vi "add set current(SubVI).vi"() -> (1 "ok or cancel":bool=TRUE, 2 "连接的字符串":string)   [LabVIEW 2019, in "Add Seq.lvlib"]
uses:
  Add Seq.lvlib
panel:
  in  "Frequency(Hz)\n(-1表示不更改频率）":dbl=-1.0 format="%#_13g"
  in  "Current Amplitude(mA)":dbl
  in  "cancel":bool
  in  "ok":bool
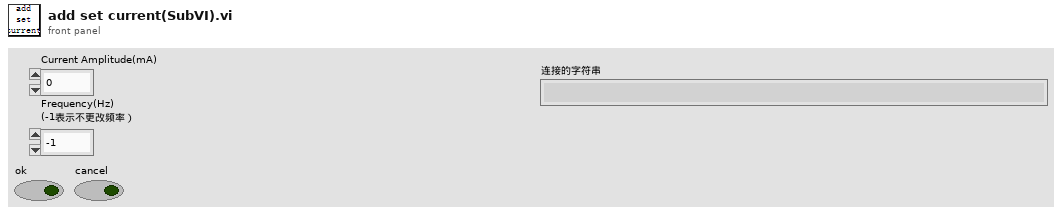
[diagram p1: front panel]
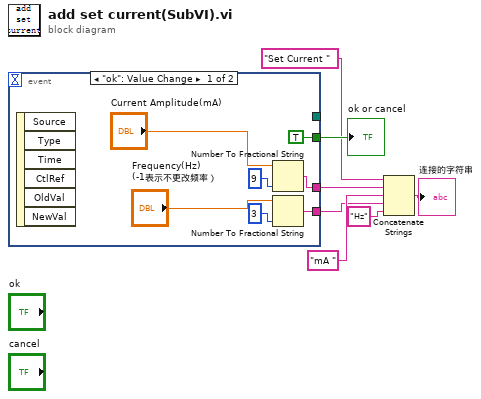
[diagram p0: block diagram]
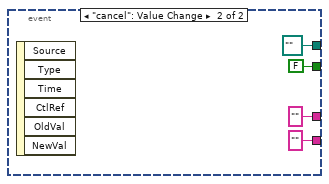
[diagram p2: hidden frame]
diagram:
  n1 = event shown="[0] \"ok\": Value Change" {
    selector: _ -> [_ _]
    dyn-events: _ -> [_ _]
    timeout: _ -> [_ _]
    tunnel: [_ path "" ("path")] -> _
    tunnel: [TRUE FALSE] -> w5
    tunnel: [w11 ""] -> w3
    tunnel: [w8 ""] -> w1
    event "ok": Value Change {
      n2 = event-data() -> ()  [unwired: 1 in, 6 out]
      n3 = Number To Fractional String(number="Current Amplitude(mA)", precision (6)=i16 9 ("精度(6)")) -> (F-format string=w11:string)  [unwired: 2 in]
      n4 = Number To Fractional String(number="Frequency(Hz)\n(-1表示不更改频率）", precision (6)=i16 3 ("精度(6)")) -> (F-format string=w8:string)  [unwired: 2 in]
    }
    event "cancel": Value Change {
      n5 = event-data() -> ()  [unwired: 1 in, 6 out]
    }
  }
  "ok or cancel" <- w5
  n6 = Concatenate Strings("Set Current " ("字符串"), w3, "mA " ("字符串"), w1, "Hz" ("字符串")) -> (→"连接的字符串":string)
